vi "WaitForAnyVI_initialize.vi"(10 "Message_command In":T1={"No. of command"=14, "Parameters"=["BLM_ManualControl.vi", "BLM Position", "Within ", "10300", "10 min"], "Address"="", "Boolean"=TRUE, "No. of line"=159, "Initial Time"=timestamp(3580981392.875361 s since 1904-01-01), "Current Time"=timestamp(0 s since 1904-01-01), "Status"="Wait for VI value ", "Sequence Ref."=refnum, "Temp check"=0, "Sequence_History"="Set Parameter BLM_ManualControl.vi, New position, 10300, Number\rSet Parameter BLM_ManualControl.vi, Run, 1, Boolean\r", "Subsequence"=[]}) -> (0 "current time":timestamp, 1 "parameters":string[](array[string]), 2 "vi reference":refnum<vi>, 3 "application reference":refnum<vi>)   [LabVIEW 2020]
uses:
  Command_Message.ctl
panel:
  out "Message_command out":T1={"No. of command"=14, "Parameters"=["BLM_ManualControl.vi", "BLM Position", "Within ", "10300", "10 min"], "Address"="", "Boolean"=TRUE, "No. of line"=159, "Initial Time"=timestamp(3580981392.875361 s since 1904-01-01), "Current Time"=timestamp(0 s since 1904-01-01), "Status"="Wait for VI value ", "Sequence Ref."=refnum, "Temp check"=0, "Sequence_History"="Set Parameter BLM_ManualControl.vi, New position, 10300, Number\rSet Parameter BLM_ManualControl.vi, Run, 1, Boolean\r", "Subsequence"=[]}
  # "VI name\nControl Name\nComparison condition\nControl to be compared\nWait time\nmachine name"
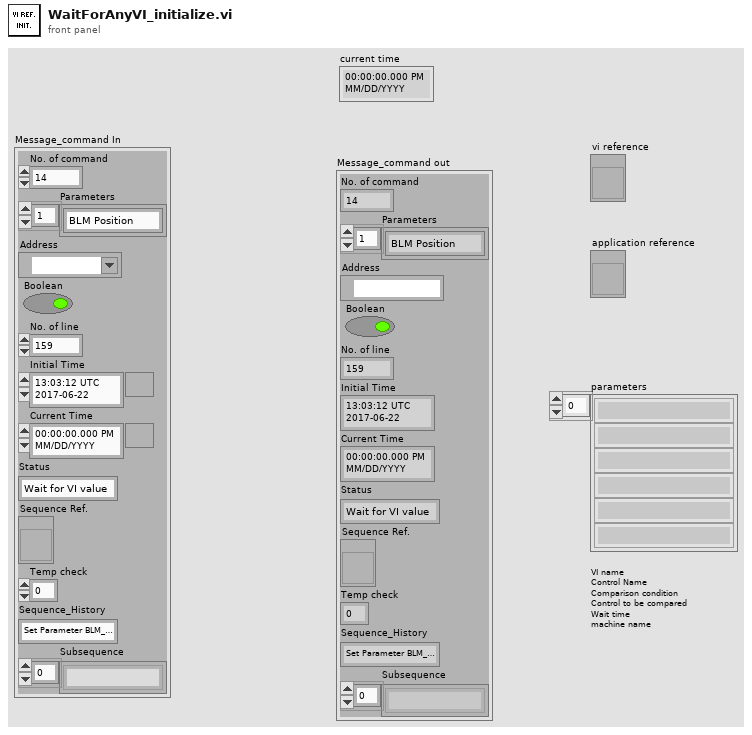
[diagram p1: front panel]
types:
  T1 = typedef "Command_Message.ctl" = cluster{"No. of command":i32, "Parameters":string[], "Address":refnum<visa-resource-name>, "Boolean":bool, "No. of line":i32, "Initial Time":timestamp, "Current Time":timestamp, "Status":string, "Sequence Ref.":refnum<vi>, "Temp check":i32, "Sequence_History":string, "Subsequence":string[]}
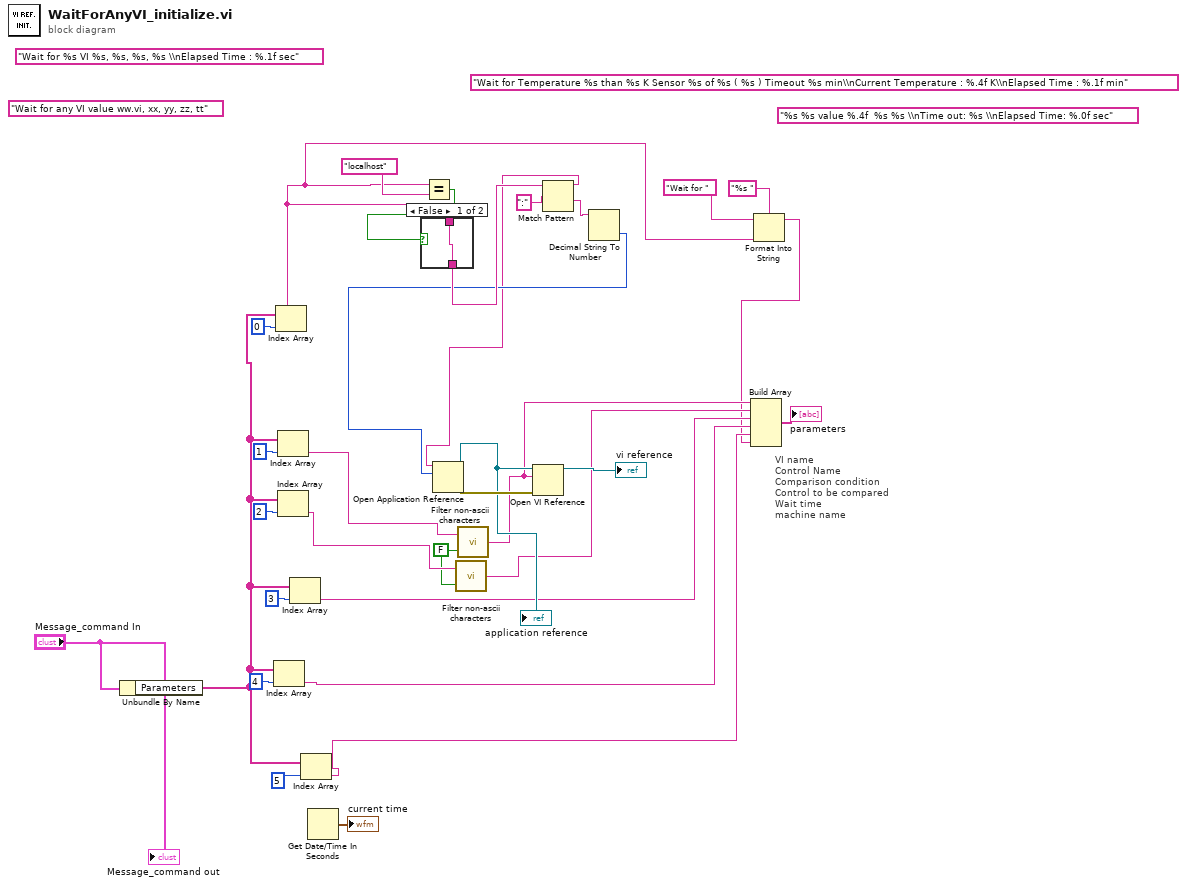
[diagram p0: block diagram]
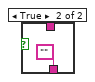
[diagram p2: hidden frame]
diagram:
  w14 = FALSE ("bypass")
  (unwired) "%s %s value %.4f  %s %s \\nTime out: %s \\nElapsed Time: %.0f sec" ("format string")
  (unwired) "Wait for Temperature %s than %s K Sensor %s of %s ( %s ) Timeout %s min\\nCurrent Temperature : %.4f K\\nElapsed Time : %.1f min"
  (unwired) "Wait for any VI value ww.vi, xx, yy, zz, tt" ("format string")
  (unwired) "Wait for %s VI %s, %s, %s, %s \\nElapsed Time : %.1f sec" ("format string")
  # "VI name\nControl Name\nComparison condition\nControl to be compared\nWait time\nmachine name"
  n1 = Unbundle By Name("Message_command In") -> ("Parameters"=w10:string[])
  n2 = Index Array(array=w10, index=4) -> (element=w7:string)
  n3 = Index Array(array=w10, index=0) -> (element=w3:string)
  n4 = Index Array(array=w10, index=1) -> (element=w15:string)
  n5 = Index Array(array=w10, index=2) -> (element=w16:string)
  n6 = Index Array(array=w10, index=3) -> (element=w6:string)
  n7 = Index Array(array=w10, index=5) -> (element=w8:string)
  n8 = Get Date/Time In Seconds() -> (seconds since 1Jan1904=→"current time":timestamp)
  n9 = Equal?(x=w3, y="localhost") -> (x = y?=w24:bool)
  n10 = case shown="False" w24 {
    tunnel: [w33 ""] -> w23
    tunnel: w3 -> [w33 _]
    frame False {
    }
    frame True {
    }
  }
  n11 = call "Filter non-ascii characters.vi"("bypass"=w14, 2:w16) -> ("output"=w12:string)
  n12 = call "Filter non-ascii characters.vi"("bypass"=w14, 2:w15) -> ("output"=w13:string)
  n13 = Match Pattern(string=w23, regular expression=":") -> (before substring=w19:string, after substring=w26:string)  [unwired: 1 in, 2 out]
  n14 = Decimal String To Number(string=w26) -> (number=w20:i32)  [unwired: 2 in, 1 out]
  n15 = Open Application Reference(10:w20, 11:w19) -> (0:w21:errorcluster, 3:w17:refnum<vi>)  [unwired: 2 in]
  "application reference" <- w17
  n16 = Open VI Reference(application reference (local)=w17, vi path=w13, error in (no error)=w21) -> (vi reference=→"vi reference":refnum<vi>)  [unwired: 3 in, 1 out]
  n17 = Format Into String(format string="%s ", initial string="Wait for " ("format string"), w3) -> (resulting string=w2:string)  [unwired: 1 in, 1 out]
  n18 = Build Array(w13, w12, w6, w7, w8, w2) -> (→"parameters":string[])
  "Message_command out" <- "Message_command In"
